vi "Prograss Bar Obtain Queue.vi"(8 "error in":errorcluster) -> (0 "error out":errorcluster, 3 "Progressbar window queue ref":T1)   [LabVIEW 2017]
uses:
  Progressbar window queue ref.ctl
  Progress bar window values input cluster.ctl
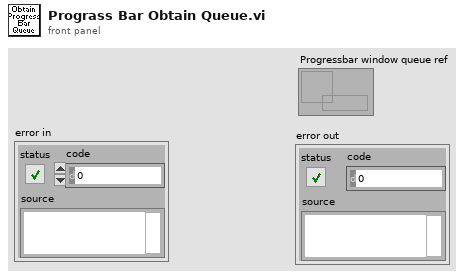
[diagram p1: front panel]
types:
  T1 = typedef "Progressbar window queue ref.ctl" = refnum<queue>
  T2 = typedef "Progress bar window values input cluster.ctl" = cluster{"Total":i32, "Current":i32, "Message in":string, "Sender":enum16{"Acquisition", "Logging", "File gen"}}
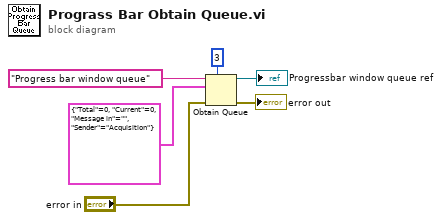
[diagram p0: block diagram]
diagram:
  n1 = Obtain Queue(max queue size (-1, unlimited)=3, name (unnamed)="Progress bar window queue", element data type=T2 {"Total"=0, "Current"=0, "Message in"="", "Sender"=enum."Acquisition"} ("Pregress bar window values input"), error in (no error)="error in") -> (queue out=→"Progressbar window queue ref":refnum<queue>, error out=→"error out":errorcluster)  [unwired: 1 in, 1 out]
